vi "readyQueues.vi"(8 "error in (no error)":errorcluster) -> (0 "error out":errorcluster, 3 "Queues":T1)   [LabVIEW 2010]
uses:
  internal_queues.ctl
  line_info.ctl
  volume_with_lines.ctl
  volume_info.ctl
  kalman_result_scaled.ctl
  projection buffers.ctl
  location3D.ctl
  spot location.ctl
  projected_volumes.ctl
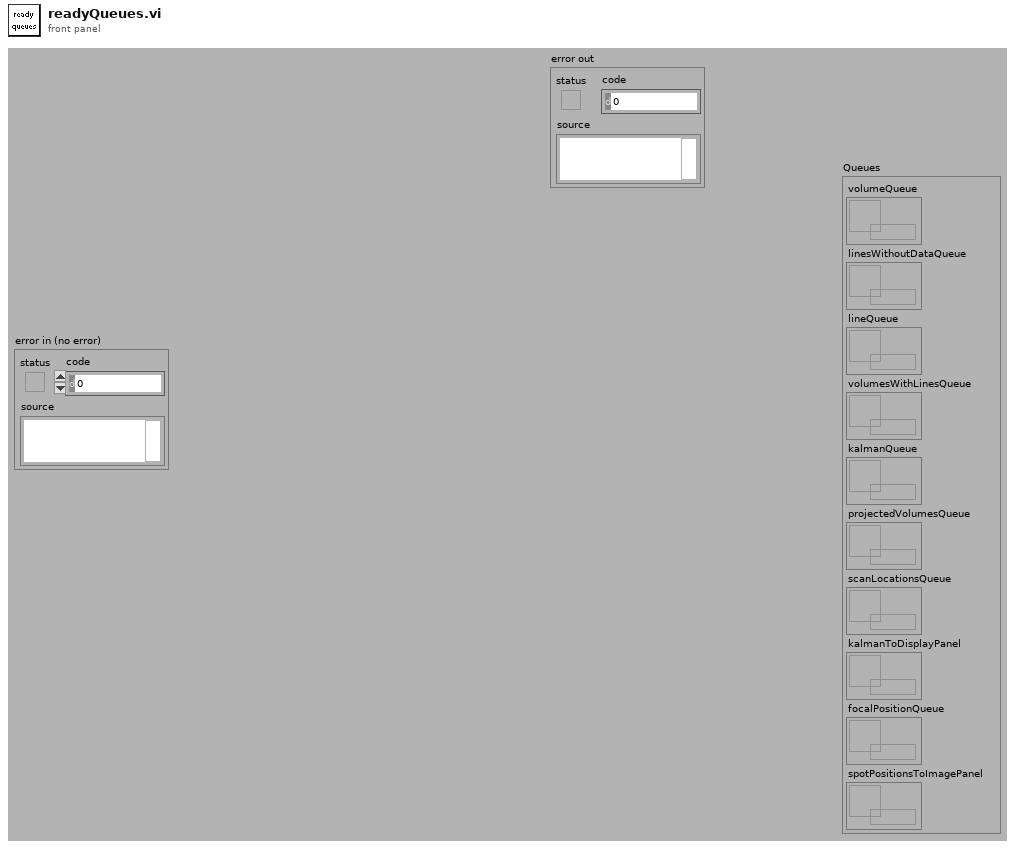
[diagram p1: front panel]
types:
  T1 = typedef "internal_queues.ctl" = cluster{"volumeQueue":refnum<queue>, "linesWithoutDataQueue":refnum<queue>, "lineQueue":refnum<queue>, "volumesWithLinesQueue":refnum<queue>, "kalmanQueue":refnum<queue>, "projectedVolumesQueue":refnum<queue>, "scanLocationsQueue":refnum<queue>, "kalmanToDisplayPanel":refnum<queue>, "focalPositionQueue":refnum<queue>, "spotPositionsToImagePanel":refnum<queue>}
  T2 = typedef "projected_volumes.ctl" = cluster{"volume info":cluster{"min x":i16, "deltaX":dbl, "num x":u32, "max x":i16, "min y":i16, "deltaY":dbl, "num y":u32, "max y":i16, "num z":u32, "num voxels":u32, "voxels read":u32, "volume num":u32}, "buffer":T3}
  T3 = typedef "projection buffers.ctl" = cluster{"xy buffer":u32[], "zx buffer":u32[], "zy buffer":u32[], "zx buffer fb only":u32[], "zy buffer fb only":u32[]}
  T4 = typedef "spot location.ctl" = cluster{"x (um)":dbl, "y (um)":dbl, "z (um)":dbl, "spot number":u8}
  T5 = typedef "location3D.ctl" = cluster{"x (um)":dbl, "y (um)":dbl, "z (um)":dbl, "time (ms)":i64}
  T6 = typedef "kalman_result_scaled.ctl" = cluster{"axis":u8, "pos":dbl, "vel":dbl, "wpe or z_piezo":dbl, "status":u32, "n photon ch 0":u32, "n photon ch 1":u32, "elapsed time":dbl}
  T7 = typedef "volume_with_lines.ctl" = cluster{"volume info":T8, "lines":T9[]}
  T8 = typedef "volume_info.ctl" = cluster{"min x":i16, "deltaX":dbl, "num x":u32, "max x":i16, "min y":i16, "deltaY":dbl, "num y":u32, "max y":i16, "num z":u32, "num voxels":u32, "voxels read":u32, "volume num":u32}
  T9 = typedef "line_info.ctl" = cluster{"start X":i16, "start Y":i16, "start Z":i16, "end X":i16, "end Y":i16, "end Z":i16, "num z":u8, "voxel data":u32[], "volume num":u32, "line number":u16, "line type":u16}
  T10 = cluster{"min x":i16, "deltaX":dbl, "num x":u32, "max x":i16, "min y":i16, "deltaY":dbl, "num y":u32, "max y":i16, "num z":u32, "num voxels":u32, "voxels read":u32, "volume num":u32}
  T11 = cluster{"queue out":refnum<queue>, "queue out":refnum<queue>, "queue out":refnum<queue>, "queue out":refnum<queue>, "queue out":refnum<queue>, "queue out":refnum<queue>, "queue out":refnum<queue>, "queue out":refnum<queue>, "queue out":refnum<queue>, "queue out":refnum<queue>}
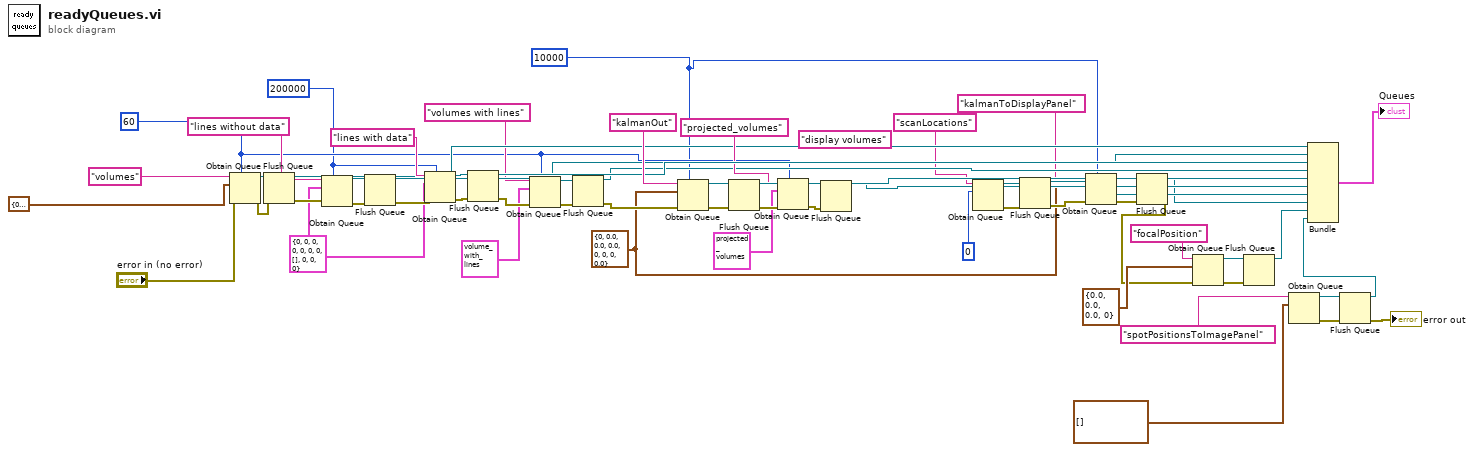
[diagram p0: block diagram]
diagram:
  w14 = 10000 ("max queue size (-1, unlimited)")
  w20 = 200000 ("max queue size (-1, unlimited)")
  w21 = 60 ("max queue size (-1, unlimited)")
  w7 = T6 {"axis"=0, "pos"=0.0, "vel"=0.0, "wpe or z_piezo"=0.0, "status"=0, "n photon ch 0"=0, "n photon ch 1"=0, "elapsed time"=0.0} ("kalman result")
  w37 = T9 {"start X"=0, "start Y"=0, "start Z"=0, "end X"=0, "end Y"=0, "end Z"=0, "num z"=0, "voxel data"=[], "volume num"=0, "line number"=0, "line type"=0} ("line status")
  (unwired) "display volumes" ("name (unnamed)")
  n1 = Obtain Queue(max queue size (-1, unlimited)=w21, name (unnamed)="volumes" ("volumes"), element data type=T10 {"min x"=0, "deltaX"=0.0, "num x"=0, "max x"=0, "min y"=0, "deltaY"=0.0, "num y"=0, "max y"=0, "num z"=0, "num voxels"=0, "voxels read"=0, "volume num"=0} ("volume info"), error in (no error)="error in (no error)") -> (queue out=w56:refnum<queue>, error out=w53:errorcluster)  [unwired: 1 in, 1 out]
  n2 = Flush Queue(queue=w56, error in (no error)=w53) -> (queue out=w40:refnum<queue>, error out=w42:errorcluster)  [unwired: 1 out]
  n3 = Obtain Queue(max queue size (-1, unlimited)=w20, name (unnamed)="lines without data", element data type=w37, error in (no error)=w42) -> (queue out=w38:refnum<queue>, error out=w41:errorcluster)  [unwired: 1 in, 1 out]
  n4 = Flush Queue(queue=w38, error in (no error)=w41) -> (queue out=w35:refnum<queue>, error out=w39:errorcluster)  [unwired: 1 out]
  n5 = Obtain Queue(max queue size (-1, unlimited)=w20, name (unnamed)="lines with data", element data type=w37, error in (no error)=w39) -> (queue out=w55:refnum<queue>, error out=w51:errorcluster)  [unwired: 1 in, 1 out]
  n6 = Flush Queue(queue=w55, error in (no error)=w51) -> (queue out=w52:refnum<queue>, error out=w31:errorcluster)  [unwired: 1 out]
  n7 = Obtain Queue(max queue size (-1, unlimited)=w21, name (unnamed)="volumes with lines", element data type=T7 {"volume info"={"min x"=0, "deltaX"=0.0, "num x"=0, "max x"=0, "min y"=0, "deltaY"=0.0, "num y"=0, "max y"=0, "num z"=0, "num voxels"=0, "voxels read"=0, "volume num"=0}, "lines"=[]} ("Cluster"), error in (no error)=w31) -> (queue out=w33:refnum<queue>, error out=w32:errorcluster)  [unwired: 1 in, 1 out]
  n8 = Flush Queue(queue=w33, error in (no error)=w32) -> (queue out=w27:refnum<queue>, error out=w30:errorcluster)  [unwired: 1 out]
  n9 = Obtain Queue(max queue size (-1, unlimited)=w14, name (unnamed)="kalmanOut", element data type=w7, error in (no error)=w30) -> (queue out=w54:refnum<queue>, error out=w49:errorcluster)  [unwired: 1 in, 1 out]
  n10 = Flush Queue(queue=w54, error in (no error)=w49) -> (queue out=w50:refnum<queue>, error out=w48:errorcluster)  [unwired: 1 out]
  n11 = Obtain Queue(max queue size (-1, unlimited)=w21, name (unnamed)="projected_volumes", element data type=T2 {"volume info"={"min x"=0, "deltaX"=0.0, "num x"=0, "max x"=0, "min y"=0, "deltaY"=0.0, "num y"=0, "max y"=0, "num z"=0, "num voxels"=0, "voxels read"=0, "volume num"=0}, "buffer"={"xy buffer"=[], "zx buffer"=[], "zy buffer"=[], "zx buffer fb only"=[], "zy buffer fb only"=[]}} ("completed volumes"), error in (no error)=w48) -> (queue out=w46:refnum<queue>, error out=w47:errorcluster)  [unwired: 1 in, 1 out]
  n12 = Flush Queue(queue=w46, error in (no error)=w47) -> (queue out=w43:refnum<queue>)  [unwired: 2 out]
  n13 = Obtain Queue(name (unnamed)="scanLocations", element data type=u32 0) -> (queue out=w25:refnum<queue>, error out=w26:errorcluster)  [unwired: 3 in, 1 out]
  n14 = Flush Queue(queue=w25, error in (no error)=w26) -> (queue out=w22:refnum<queue>, error out=w17:errorcluster)  [unwired: 1 out]
  n15 = Obtain Queue(max queue size (-1, unlimited)=w14, name (unnamed)="kalmanToDisplayPanel", element data type=w7, error in (no error)=w17) -> (queue out=w19:refnum<queue>, error out=w18:errorcluster)  [unwired: 1 in, 1 out]
  n16 = Flush Queue(queue=w19, error in (no error)=w18) -> (queue out=w15:refnum<queue>, error out=w9:errorcluster)  [unwired: 1 out]
  n17 = Obtain Queue(name (unnamed)="focalPosition", element data type=T5 {"x (um)"=0.0, "y (um)"=0.0, "z (um)"=0.0, "time (ms)"=0} ("location"), error in (no error)=w9) -> (queue out=w13:refnum<queue>, error out=w12:errorcluster)  [unwired: 2 in, 1 out]
  n18 = Flush Queue(queue=w13, error in (no error)=w12) -> (queue out=w8:refnum<queue>)  [unwired: 2 out]
  n19 = Obtain Queue(name (unnamed)="spotPositionsToImagePanel", element data type=T4[] []) -> (queue out=w5:refnum<queue>, error out=w4:errorcluster)  [unwired: 3 in, 1 out]
  n20 = Flush Queue(queue=w5, error in (no error)=w4) -> (queue out=w3:refnum<queue>, error out=→"error out":errorcluster)  [unwired: 1 out]
  n21 = Bundle("queue out"=w40, "queue out"=w35, "queue out"=w52, "queue out"=w27, "queue out"=w50, "queue out"=w43, "queue out"=w22, "queue out"=w15, "queue out"=w8, "queue out"=w3) -> (→"Queues":T11)  [unwired: 1 in]
